vi "Develop.vi"() -> ()   [LabVIEW 2019]
panel:
  out "Boolean 2":bool
  out "Boolean":bool
  out "Numeric 2":dbl
  in  "Numeric2":dbl
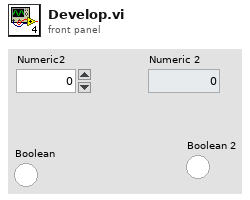
[diagram p1: front panel]
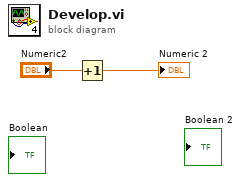
[diagram p0: block diagram]
diagram:
  n1 = Increment(x="Numeric2") -> (x+1=→"Numeric 2":dbl)
